vi "WriteToCSV_FVIR.vi"(6 "StartTime":string, 10 "PLC Data Out":T1, 11 "file path (dialog if empty)":path) -> ()   [LabVIEW 2020, in "WritingDataFile.lvlib"]
uses:
  WritingDataFile.lvlib
  Modbus/Modbus PLC Data All.ctl
  Modbus/Modbus FVIR Control.ctl
  Modbus/Modbus LDO Control.ctl
  Data to Save.ctl
  <vilib>/Utility/file.llb/Write Delimited Spreadsheet (string).vi
panel:
  out "resulting string":string
  out "Time Difference (HH:MM:SS)":dbl format="%<%H:%M:%S>t"
  out "Time Difference (Seconds)":dbl
  out "Data to write to csv":string[](array[string])
  out "file path (dialog if empty) 2":path
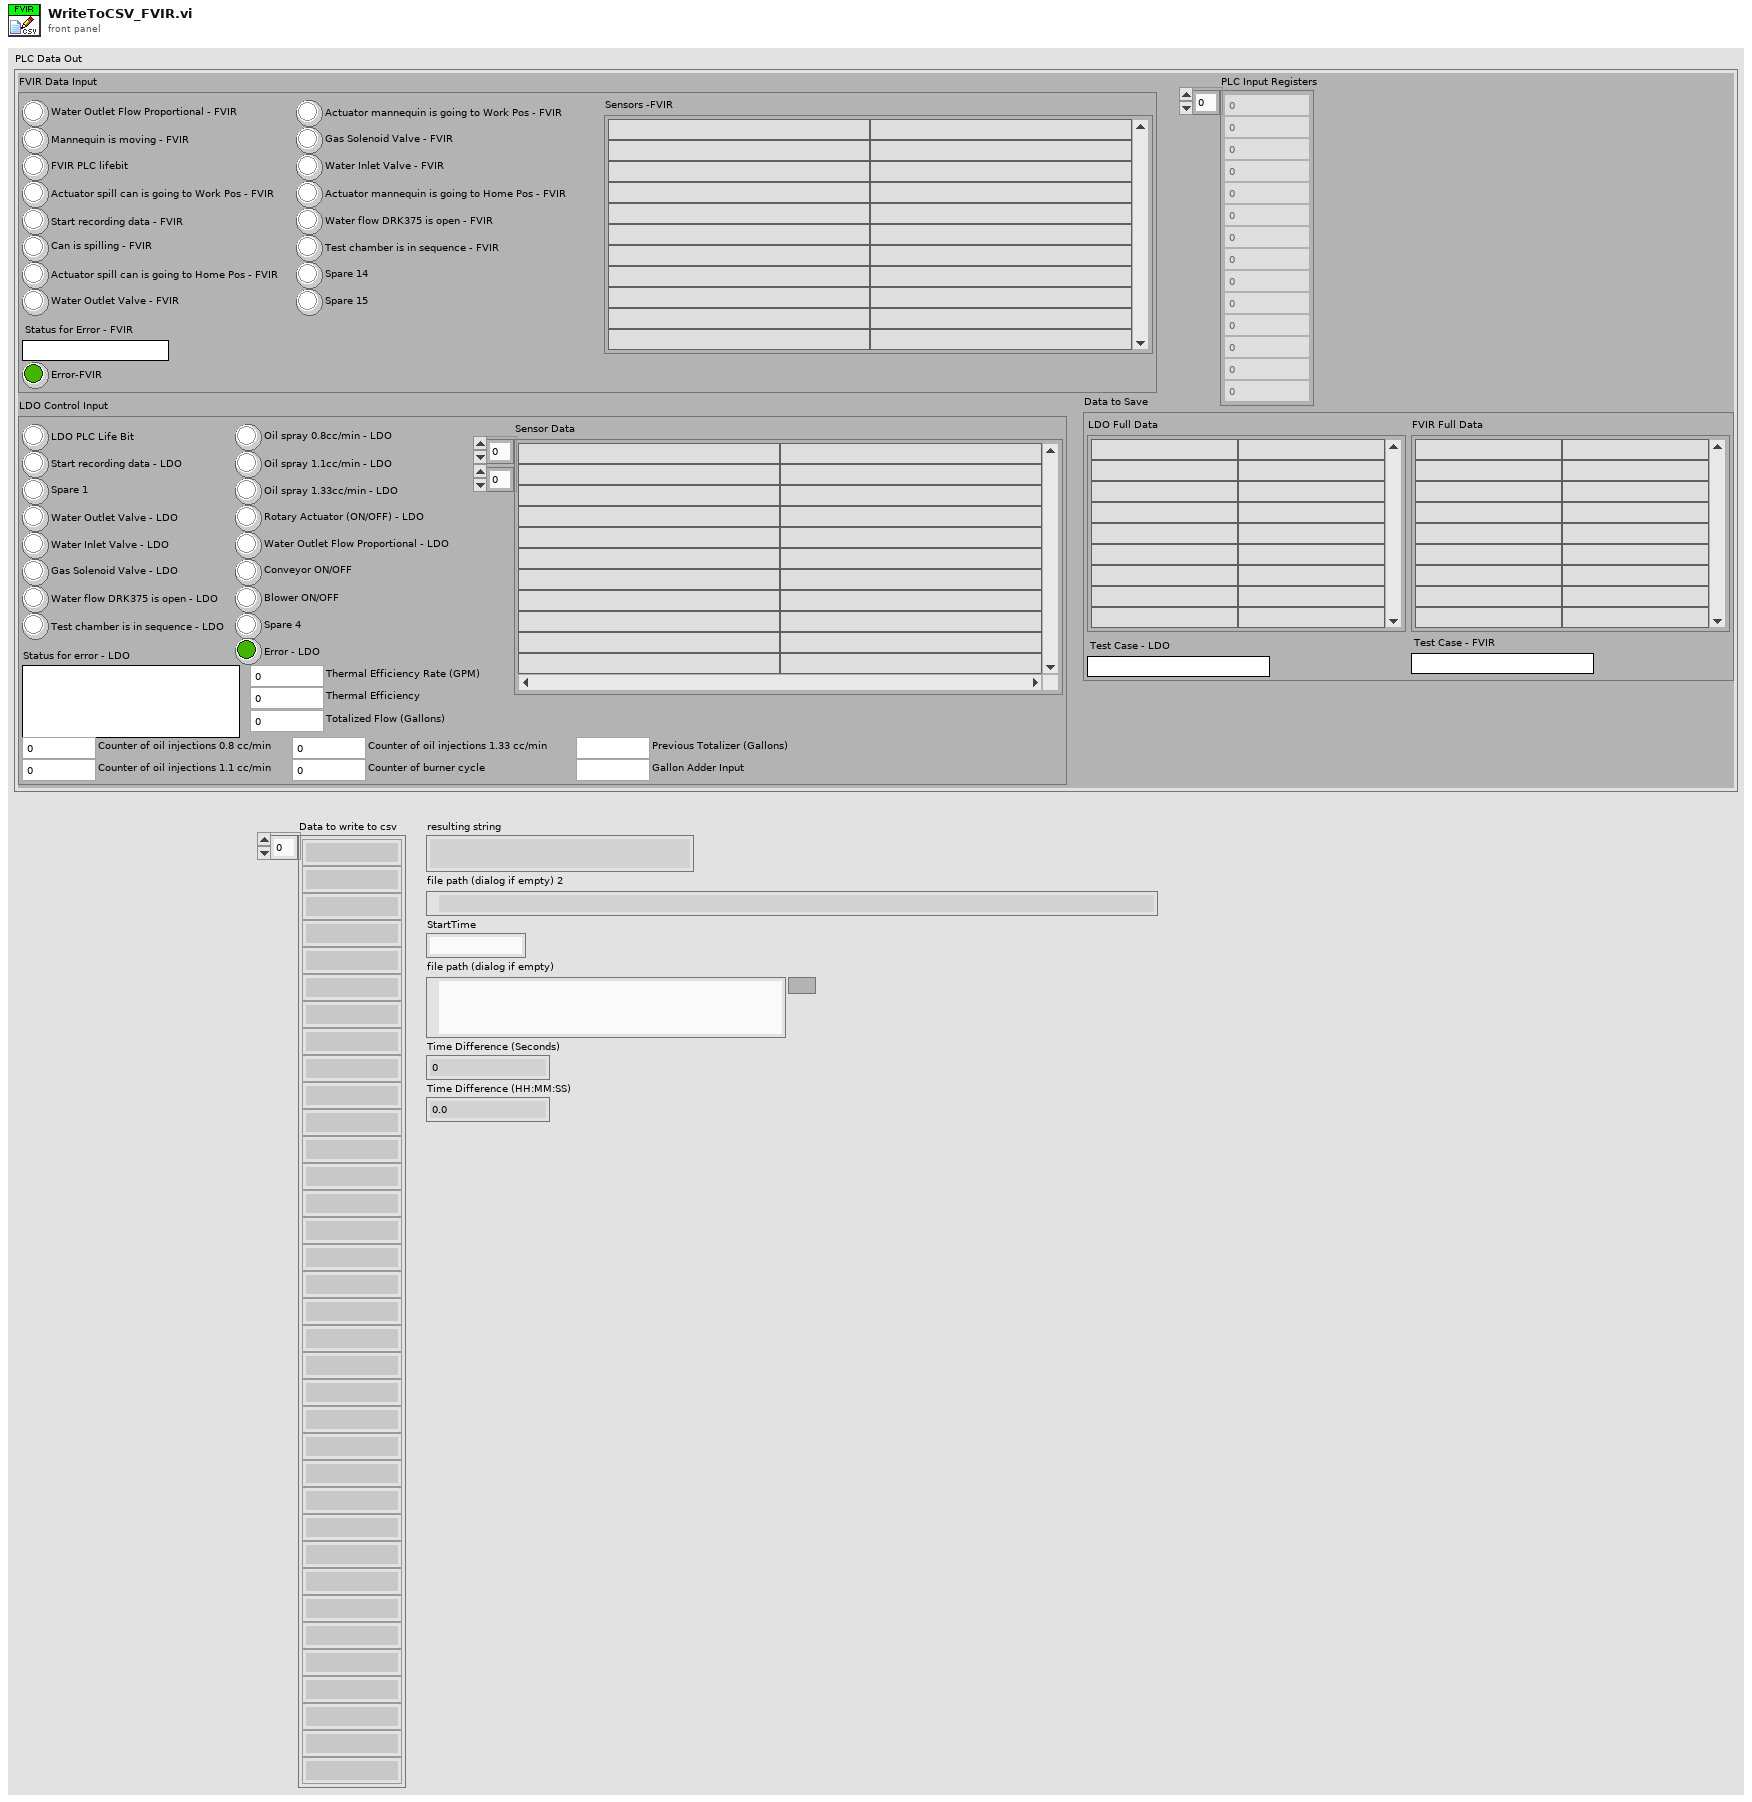
[diagram p1: front panel]
types:
  T1 = typedef "Modbus PLC Data All.ctl" = cluster{"FVIR Data Input":T2, "LDO Control Input":T3, "PLC Input Registers":i16[], "Data to Save":T4}
  T2 = typedef "Modbus FVIR Control.ctl" = cluster{"Spare 15":bool, "Spare 14":bool, "Actuator mannequin is going to Work Pos - FVIR":bool, "Actuator mannequin is going to Home Pos - FVIR":bool, "Test chamber is in sequence - FVIR ":bool, "Water flow DRK375 is open - FVIR":bool, "Gas Solenoid Valve - FVIR":bool, "Water Inlet Valve - FVIR":bool, "Water Outlet Flow Proportional - FVIR":bool, "Start recording data - FVIR":bool, "Actuator spill can is going to Work Pos - FVIR":bool, "Actuator spill can is going to Home Pos - FVIR":bool, "Water Outlet Valve - FVIR":bool, "Can is spilling - FVIR":bool, "Mannequin is moving - FVIR":bool, "FVIR PLC lifebit":bool, "Status for Error - FVIR":string, "Error-FVIR":bool, "Sensors -FVIR":string[][]}
  T3 = typedef "Modbus LDO Control.ctl" = cluster{"LDO PLC Life Bit":bool, "Start recording data - LDO":bool, "Spare 1":bool, "Water Outlet Valve - LDO":bool, "Water Inlet Valve - LDO":bool, "Gas Solenoid Valve - LDO":bool, "Water flow DRK375 is open - LDO":bool, "Test chamber is in sequence - LDO":bool, "Oil spray 0.8cc/min - LDO":bool, "Oil spray 1.1cc/min - LDO":bool, "Oil spray 1.33cc/min - LDO":bool, "Rotary Actuator (ON/OFF) - LDO":bool, "Water Outlet Flow Proportional - LDO":bool, "Conveyor ON/OFF":bool, "Blower ON/OFF":bool, "Spare 4":bool, "Status for error - LDO":string, "Error - LDO":bool, "Sensor Data":string[][], "Thermal Efficiency Rate (GPM)":dbl, "Thermal Efficiency":dbl, "Totalized Flow (Gallons)":dbl, "Counter of oil injections 1.33 cc/min":u16, "Counter of burner cycle":u16, "Counter of oil injections 1.1 cc/min":u16, "Counter of oil injections 0.8 cc/min":u16, "Previous Totalizer (Gallons)":dbl, "Gallon Adder Input":dbl}
  T4 = typedef "Data to Save.ctl" = cluster{"LDO Full Data":string[][], "FVIR Full Data":string[][], "Test Case - FVIR":string, "Test Case - LDO":string}
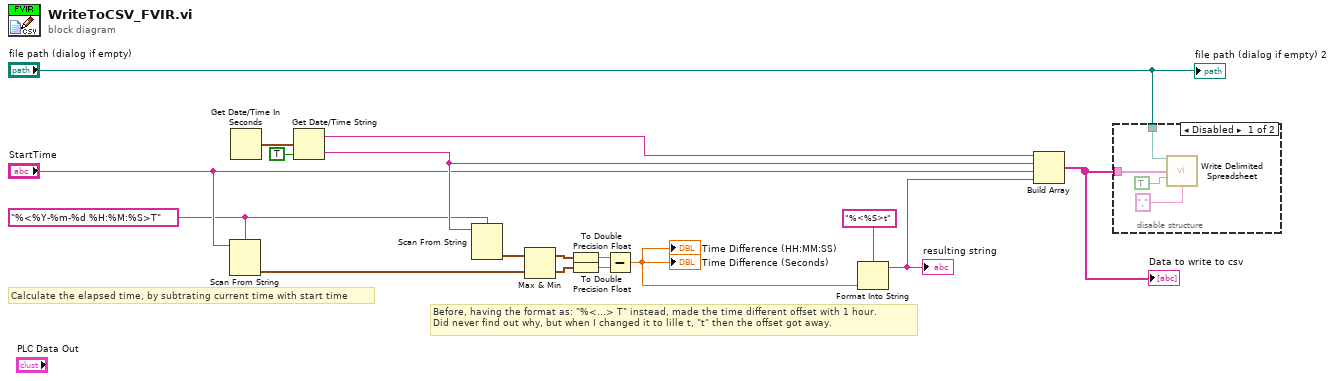
[diagram p0: block diagram]
diagram:
  w1 = "%<%Y-%m-%d %H:%M:%S>T" ("format string")
  # "Before, having the format as: \"%<...> T\" instead, made the time different offset with 1 hour. \nDid never find out why, but when I changed it to lille t, \"t\" then the offset got away."
  # "Calculate the elapsed time, by subtrating current time with start time"
  n1 = Scan From String(format string=w1, input string="StartTime") -> (output 1=w12:timestamp)  [unwired: 3 in, 3 out]
  n2 = Get Date/Time In Seconds() -> (seconds since 1Jan1904=w17:timestamp)
  n3 = Get Date/Time String(seconds (now)=w17, want seconds? (F)=TRUE) -> (date string=w5:string, time string=w4:string)  [unwired: 1 in]
  n4 = Scan From String(format string=w1, input string=w4) -> (output 1=w13:timestamp)  [unwired: 3 in, 3 out]
  n5 = Max & Min(x=w13, y=w12) -> (max(x,y)=w11:timestamp, min(x,y)=w10:timestamp)
  n6 = To Double Precision Float(number=w11) -> (double precision float=w9:dbl)
  n7 = To Double Precision Float(number=w10) -> (double precision float=w8:dbl)
  n8 = Subtract(x=w9, y=w8) -> (x-y=w6:dbl)
  "Time Difference (Seconds)" <- w6
  "Time Difference (HH:MM:SS)" <- w6
  n9 = Format Into String(format string="%<%S>t", w6) -> (resulting string=w2:string)  [unwired: 2 in, 1 out]
  "resulting string" <- w2
  n10 = Build Array(w5, w4, "StartTime", w2) -> (w15:string[])
  "Data to write to csv" <- w15
  n11 = disable-structure shown="Disabled" {
    disable-tunnel: w15 -> [w21 _]
    disable-tunnel: "file path (dialog if empty)" -> [w20 _]
    frame Disabled {
      n12 = call-poly <vilib>:"Write Delimited Spreadsheet.vi"("file path (dialog if empty)"=w20, "1D data"=w21, "append to file? (new file:F)"=TRUE, "delimiter (\\t)"="," ("delimiter (\\t)")) -> ()  [unwired: 10 in, 2 out]
    }
    frame Enabled {
    }
  }
  "file path (dialog if empty) 2" <- "file path (dialog if empty)"
